vi "Track_Tip_DAQ.vi"(8 "error in":errorcluster, 11 "physical channels":tag="Dev4/ai0:3") -> (0 "error out":errorcluster, 3 "data":dbl[][](array[numeric]))   [LabVIEW 2016]
uses:
  <vilib>/DAQmx/read.llb/DAQmx Read (Analog 2D DBL NChan NSamp).vi
  <vilib>/DAQmx/create/channels.llb/DAQmx Create Channel (AI-Voltage-Basic).vi
  <vilib>/DAQmx/configure/timing.llb/DAQmx Timing (Sample Clock).vi
  <vilib>/DAQmx/miscellaneous.llb/DAQmx Fill In Error Info.vi
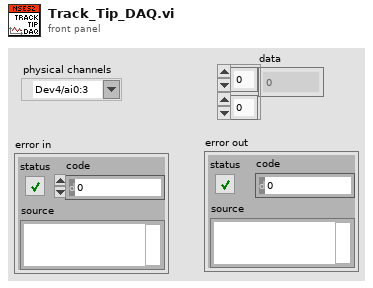
[diagram p1: front panel]
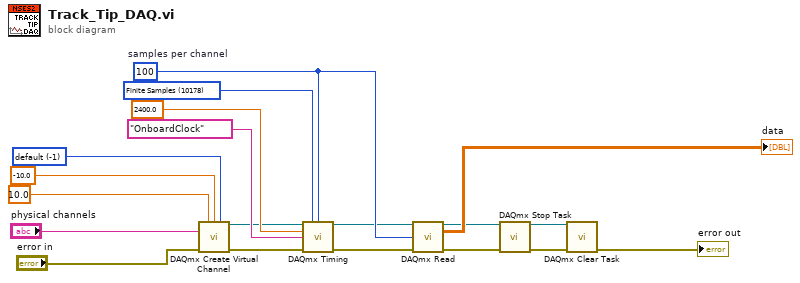
[diagram p0: block diagram]
diagram:
  w15 = 100  # samples per channel
  w8 = 10178 items=["Finite Samples"=10178, "Continuous Samples"=10123, "Hardware Timed Single Point"=12522] ("sample mode")
  w7 = -1 items=["default"=-1, "RSE"=10083, "NRSE"=10078, "Differential"=10106, "Pseudodifferential"=12529] ("input terminal configuration")
  n1 = call-poly <vilib>:"DAQmx Create Virtual Channel.vi"("maximum value"=10.0, "minimum value"=-10.0, "input terminal configuration"=w7, "physical channels"="physical channels", "error in"="error in") -> ("task out"=w9:refnum<k21>, "error out"=w1:errorcluster)  [unwired: 9 in]
  n2 = call-poly <vilib>:"DAQmx Timing.vi"("task/channels in"=w9, "sample mode"=w8, "samples per channel"=w15, "rate"=2400.0, "source"=tag "OnboardClock", "error in"=w1) -> ("task out"=w10:refnum<k21>, "error out"=w2:errorcluster)  [unwired: 8 in]
  n3 = call-poly <vilib>:"DAQmx Read.vi"("task/channels in"=w10, "number of samples per channel"=w15, "error in"=w2) -> ("task out"=w13:refnum<k21>, "data"=→"data":dbl[][], "error out"=w14:errorcluster)  [unwired: 10 in]
  n4 = call <vilib>:"DAQmx Stop Task.vi"("task/channels in"=w13, "error in"=w14) -> ("task out"=w11:refnum<k21>, "error out"=w3:errorcluster)  [unwired: 12 in]
  n5 = call <vilib>:"DAQmx Clear Task.vi"("task in"=w11, "error in"=w3) -> ("error out"=→"error out":errorcluster)  [unwired: 13 in]
